vi "DownConvert AssertEventData.vi"(10 "Assert Event Data (Extended)":T2={"name"="", "passed"=FALSE, "call-chain"=[], "test-error"={"status"=FALSE, "code"=0, "source"=""}, "timestamp"=timestamp(0 s since 1904-01-01), "assert-id"="", "test-id"="", "time"=-1.0, "message"="", "properties"=variant, "measurements"=variant, "user-defined"=variant}) -> (2 "Assert Event Data":T1={"Name"="", "Passed"=FALSE, "Call Chain"=[], "Test Error"={"status"=FALSE, "code"=0, "source"=""}, "Time Stamp"=timestamp(0 s since 1904-01-01), "Unique Assert ID"="", "Test ID"="", "Execution time (s)"=-1.0, "Verbose Explanation"=""})   [LabVIEW 2020, in "Caraya.lvlib" / "Test Result.lvclass"]
uses:
  Test Result.lvclass
  Assert Event Data (Extended).ctl
  Assert Event Data.ctl
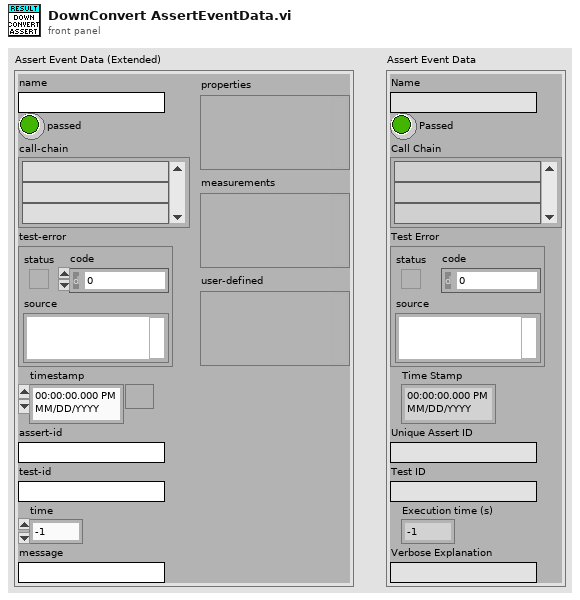
[diagram p1: front panel]
types:
  T1 = typedef "Caraya.lvlib/Test Result.lvclass/Assert Event Data.ctl" = cluster{"Name":string, "Passed":bool, "Call Chain":string[], "Test Error":errorcluster, "Time Stamp":timestamp, "Unique Assert ID":string, "Test ID":string, "Execution time (s)":dbl, "Verbose Explanation":string}
  T2 = typedef "Caraya.lvlib/Test Result.lvclass/Assert Event Data (Extended).ctl" = cluster{"name":string, "passed":bool, "call-chain":string[], "test-error":errorcluster, "timestamp":timestamp, "assert-id":string, "test-id":string, "time":dbl, "message":string, "properties":variant, "measurements":variant, "user-defined":variant}
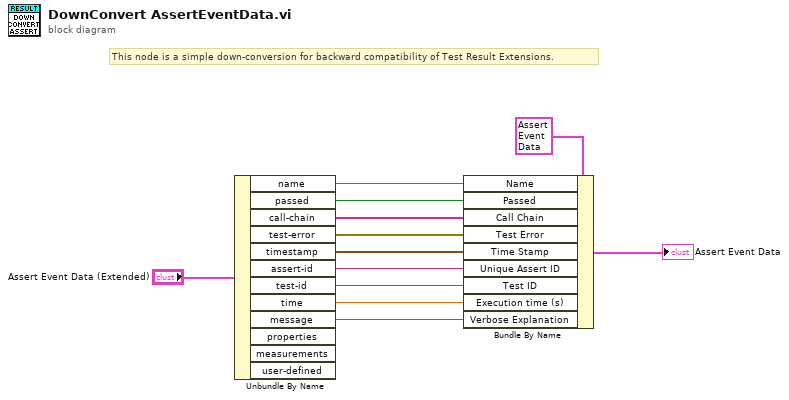
[diagram p0: block diagram]
diagram:
  # "This node is a simple down-conversion for backward compatibility of Test Result Extensions."
  n1 = Unbundle By Name("Assert Event Data (Extended)") -> ("name"=w10:string, "passed"=w9:bool, "call-chain"=w8:string[], "test-error"=w7:errorcluster, "timestamp"=w6:timestamp, "assert-id"=w5:string, "test-id"=w4:string, "time"=w3:dbl, "message"=w2:string)  [unwired: 3 out]
  n2 = Bundle By Name(cluster=T1 {"Name"="", "Passed"=FALSE, "Call Chain"=[], "Test Error"={"status"=FALSE, "code"=0, "source"=""}, "Time Stamp"=timestamp(0 s since 1904-01-01), "Unique Assert ID"="", "Test ID"="", "Execution time (s)"=-1.0, "Verbose Explanation"=""} ("Test Event"), "Name"=w10, "Passed"=w9, "Call Chain"=w8, "Test Error"=w7, "Time Stamp"=w6, "Unique Assert ID"=w5, "Test ID"=w4, "Execution time (s)"=w3, "Verbose Explanation"=w2) -> (→"Assert Event Data":T1)
